vi "HGCROC Glue Testing.vi"   [LabVIEW 2020]
uses:
  Classes/Workspace/Carrier Tray/Assembly Tray.lvclass
  Classes/Routine/Dispense/CAD Dispense/8 Inch CAD Dispense.lvclass
  Classes/Routine/Secure Syringe/SecureRelease Syringe.lvclass
  Classes/Workspace/Carrier Tray/Syringe Space/Syringe Space.lvclass
  Classes/Routine/Secure Syringe/SecureRelease Syringe.lvclass/SecureRelease Syringe.ctl
  Classes/Routine/Secure Syringe/Write Type.vi
  Classes/Controller/Controller.lvclass
types:
  T1 = typedef "Controller.lvclass/Controllers.ctl" = cluster{"I-O.lvclass":refnum<class "I-O.lvclass">, "Dispenser.lvclass":refnum<class "Dispenser.lvclass">, "Gantry":refnum<k24>}
  T2 = typedef "Fixture.lvclass/Workspace.ctl" = cluster{"XYZTheta":dbl[], "Workspace Valve":i32, "Workspace Sensor":i32}
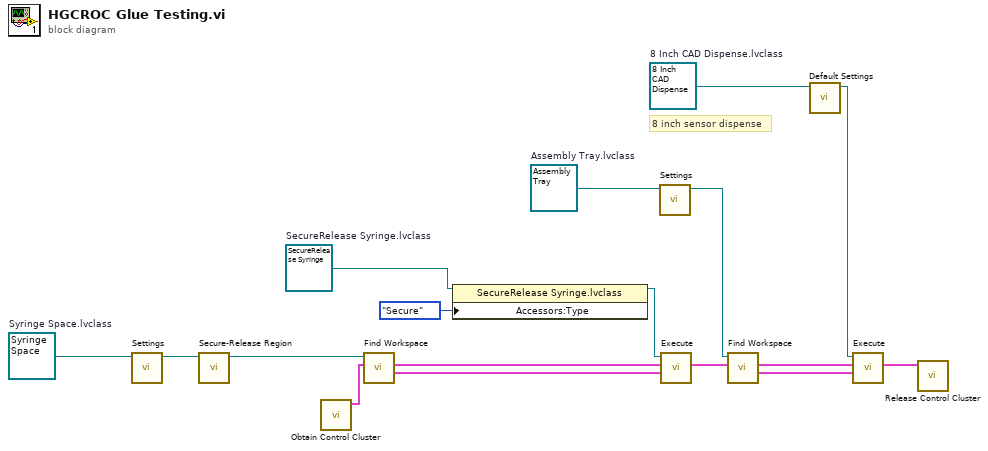
[diagram p0: block diagram]
diagram:
  w3 = refnum<class "Syringe Space.lvclass"> refnum  # Syringe Space.lvclass
  w11 = refnum<class "SecureRelease Syringe.lvclass"> refnum  # SecureRelease Syringe.lvclass
  w16 = refnum<class "8 Inch CAD Dispense.lvclass"> refnum  # 8 Inch CAD Dispense.lvclass
  w17 = refnum<class "Assembly Tray.lvclass"> refnum  # Assembly Tray.lvclass
  # "8 inch sensor dispense"
  n1 = call-dynamic "Settings.vi"("Syringe Space in"=w3) -> ("Syringe Space out"=w7:refnum<class "Syringe Space.lvclass">)  [unwired: 9 in, 1 out]
  n2 = call-dynamic "Secure-Release Region.vi"("Carrier Tray in"=w7) -> ("Carrier Tray out"=w6:refnum<class "Syringe Space.lvclass">)  [unwired: 8 in, 2 out]
  n3 = call "Obtain Control Cluster.vi"() -> ("Control Out"=w9:T1)  [unwired: 11 in]
  n4 = call-dynamic "Find Workspace.vi"("Control In"=w9, "Carrier Tray in"=w6) -> ("Workspace"=w5:T2, "Control Out"=w8:T1)  [unwired: 6 in, 2 out]
  n5 = property class="SecureRelease Syringe.lvclass"(reference=w11, "Accessors:Type"=enum16{"Secure", "Remove"}."Secure" ("Type")) -> (reference out=w4:refnum<class "SecureRelease Syringe.lvclass">)  [unwired: 1 in, 1 out]
  n6 = call-dynamic "Settings.vi"("Assembly Tray In"=w17) -> ("Assembly Tray Out"=w2:refnum<class "Assembly Tray.lvclass">)  [unwired: 9 in, 1 out]
  n7 = call-dynamic "Execute.vi"("Workspace"=w5, "Control In"=w8, "Secure Syringe in"=w4) -> ("Control Out"=w1:T1)  [unwired: 6 in, 2 out]
  n8 = call-dynamic "Find Workspace.vi"("Control In"=w1, "Carrier Tray in"=w2) -> ("Workspace"=w14:T2, "Control Out"=w13:T1)  [unwired: 6 in, 2 out]
  n9 = call-dynamic "Default Settings.vi"("8 Inch CAD Dispense in"=w16) -> ("8 Inch CAD Dispense out"=w15:refnum<class "8 Inch CAD Dispense.lvclass">)  [unwired: 9 in, 1 out]
  n10 = call-dynamic "Execute.vi"("Workspace"=w14, "Control In"=w13, "Dispense in"=w15) -> ("Control Out"=w12:T1)  [unwired: 6 in, 2 out]
  n11 = call "Release Control Cluster.vi"("output cluster"=w12) -> ()  [unwired: 11 in]
